vi "Temperature Conversions.vi"() -> ()   [LabVIEW 2014]
panel:
  in  "stop":bool
  out "Converted Temperature":dbl
  in  "Temperature to Convert":dbl
  in  "Enum":T1(ring)
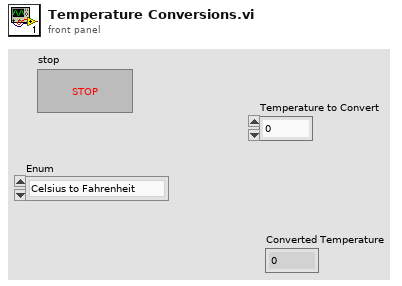
[diagram p1: front panel]
types:
  T1 = enum16{"Celsius to Fahrenheit", "Fahrenheit to Celsius", "Celsius to Kelvin", "Fahrenheit to Kelvin"}
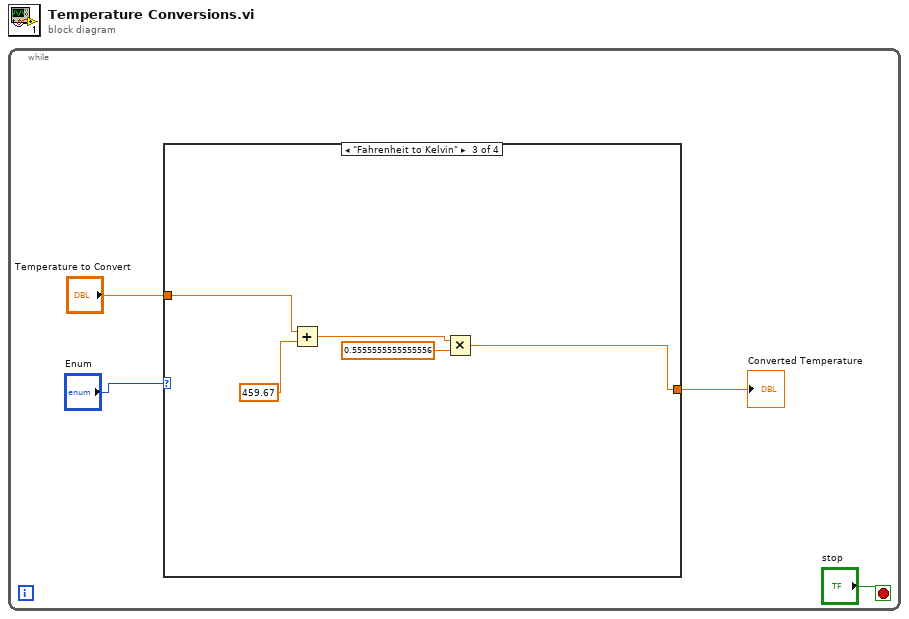
[diagram p0: block diagram]
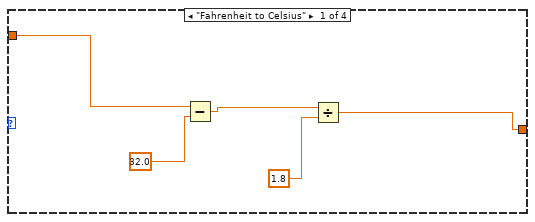
[diagram p2: hidden frame]
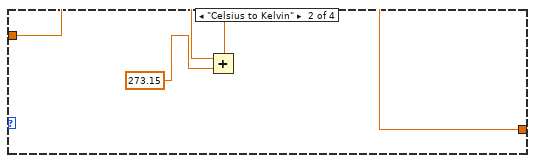
[diagram p3: hidden frame]
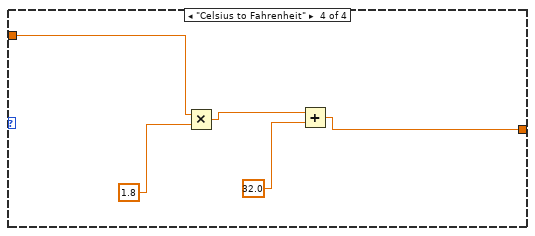
[diagram p4: hidden frame]
diagram:
  n1 = while {
    stop <- "stop" stop-if-true
    n2 = case shown="\"Fahrenheit to Kelvin\"" "Enum" {
      tunnel: "Temperature to Convert" -> [w9 w12 w16 w20]
      tunnel: [w5 w11 w13 w18] -> w2
      frame "Fahrenheit to Celsius" {
        n3 = Subtract(x=w9, y=32.0) -> (x-y=w6:dbl)
        n4 = Divide(x=w6, y=1.8) -> (x/y=w5:dbl)
      }
      frame "Celsius to Kelvin" {
        n5 = Add(x=w12, y=273.15) -> (x+y=w11:dbl)
      }
      frame "Fahrenheit to Kelvin" {
        n6 = Add(x=w16, y=459.67) -> (x+y=w14:dbl)
        n7 = Multiply(x=w14, y=0.5555555555555556) -> (x*y=w13:dbl)
      }
      frame "Celsius to Fahrenheit" {
        n8 = Multiply(x=w20, y=1.8) -> (x*y=w21:dbl)
        n9 = Add(x=w21, y=32.0) -> (x+y=w18:dbl)
      }
    }
    "Converted Temperature" <- w2
  }
